vi "Blink_SDK_example.vi"() -> ()   [LabVIEW 2010]
uses:
  Blink_C_wrapper.dll
  ImageGen.dll
panel:
  out "ImgData 2":u8[](array[numeric])
  in  "Wait Timer":dbl
  out "Use External Triggers":bool
  out "BoardNum":i32
  out "ImgData":u8[](array[numeric])
  # "PCIe  LabVIEWSDK"
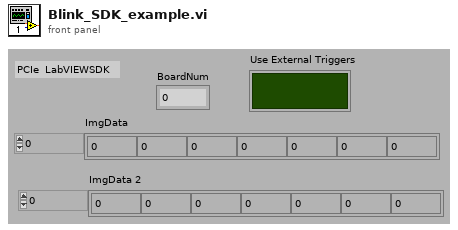
[diagram p1: front panel]
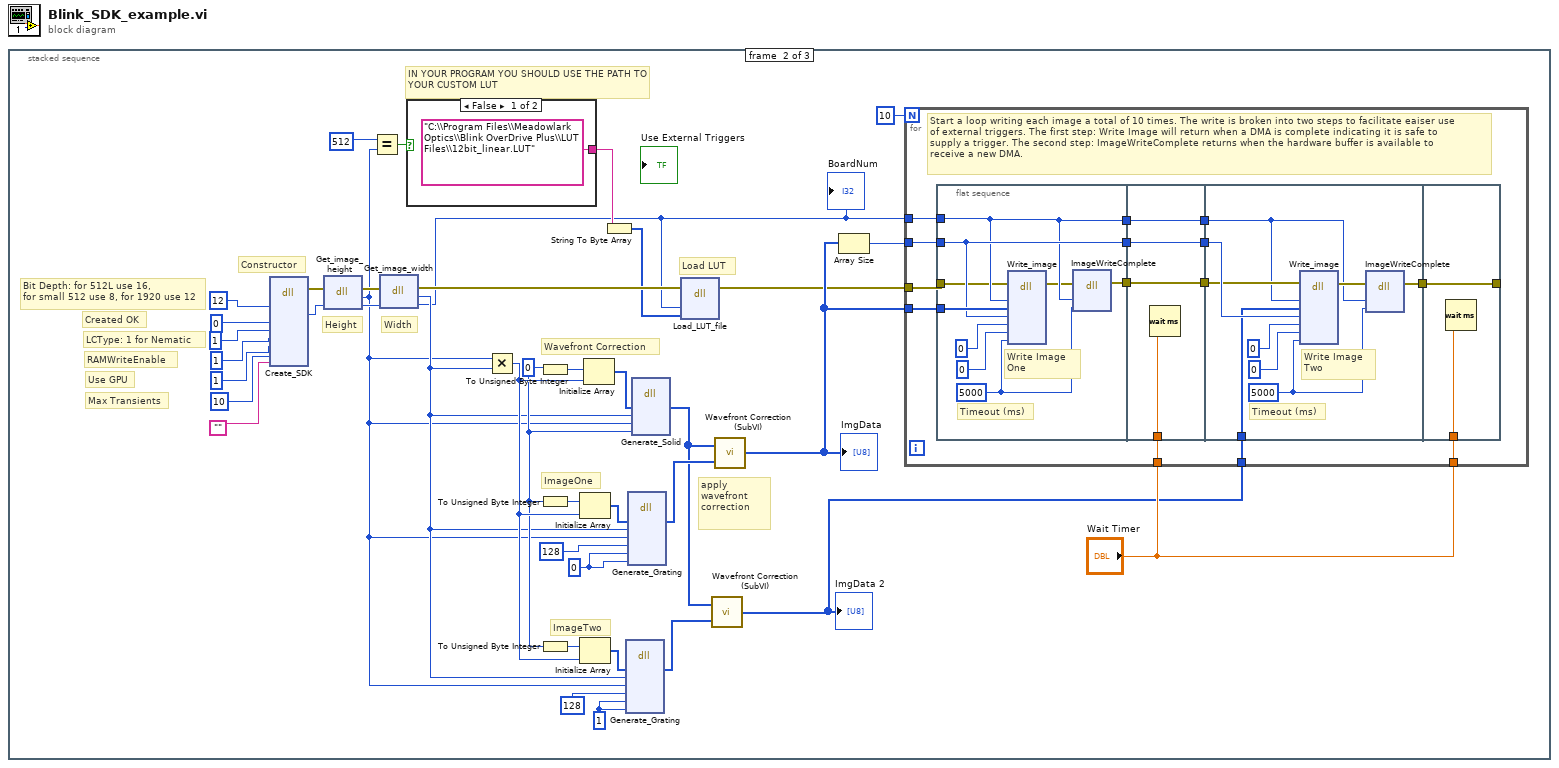
[diagram p0: block diagram]
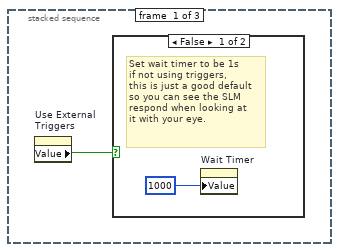
[diagram p2: hidden frame]
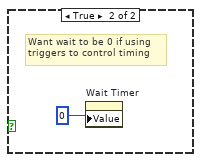
[diagram p3: hidden frame]
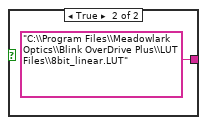
[diagram p4: hidden frame]
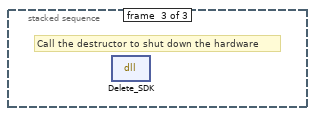
[diagram p5: hidden frame]
diagram:
  n1 = stacked-sequence {
    frame #0 {
      n2 = property on="Use External \nTriggers" class="Bool (strict)"() -> ("Value"=w1:bool)  [unwired: 2 in, 2 out]
      n3 = case shown="False" w1 {
        frame False {
          # "Set wait timer to be 1s \nif not using triggers,\nthis is just a good default \nso you can see the SLM \nrespond when looking at \nit with your eye."
          n4 = property on="Wait Timer" class="DigNum (strict)"("Value"=1000) -> ()  [unwired: 2 in, 2 out]
        }
        frame True {
          # "Want wait to be 0 if using \ntriggers to control timing"
          n5 = property on="Wait Timer" class="DigNum (strict)"("Value"=0) -> ()  [unwired: 2 in, 2 out]
        }
      }
    }
    frame #1 {
      w20 = 1
      w22 = 0
      w25 = 0
      # "IN YOUR PROGRAM YOU SHOULD USE THE PATH TO YOUR CUSTOM LUT"
      # "Load LUT"
      # "ImageTwo"
      # "ImageOne"
      # "Wavefront Correction"
      # "Width"
      # "Height"
      # "apply wavefront\ncorrection"
      # "Created OK"
      # "Max Transients"
      # "Use GPU"
      # "RAMWriteEnable"
      # "Bit Depth: for 512L use 16, \nfor small 512 use 8, for 1920 use 12"
      # "LCType: 1 for Nematic"
      # "Constructor"
      n6 = dll-call lib="C:/Program Files/Meadowlark Optics/Blink OverDrive Plus/SDK/Blink_C_wrapper.dll" fn="Create_SDK"("SLM_bit_depth"=12, "constructed_ok"=0, "is_nematic_type"=1, "RAM_write_enable"=1, "use_GPU_if_available"=1, "max_transient_frames"=10, "static_regional_lut_file"="") -> (error out=w5:errorcluster, "n_boards_found"=w4:u64)  [unwired: 12 in, 1 out]
      n7 = dll-call lib="C:/Program Files/Meadowlark Optics/Blink OverDrive Plus/SDK/Blink_C_wrapper.dll" fn="Get_image_height"(error in=w5, "Board"=w4) -> (error out=w31:errorcluster, "return type"=w9:i32, "Board"=w32:u32)  [unwired: 2 in, 1 out]
      n8 = Equal?(x=512, y=w9) -> (x = y?=w11:bool)
      n9 = dll-call lib="C:/Program Files/Meadowlark Optics/Blink OverDrive Plus/SDK/Blink_C_wrapper.dll" fn="Get_image_width"(error in=w31, "Board"=w32) -> (error out=w12:errorcluster, "return type"=w18:i32, "Board"=w6:u32)  [unwired: 2 in, 1 out]
      "BoardNum" <- w6
      n10 = case shown="False" w11 {
        tunnel: ["C:\\Program Files\\Meadowlark Optics\\Blink OverDrive Plus\\LUT Files\\12bit_linear.LUT" "C:\\Program Files\\Meadowlark Optics\\Blink OverDrive Plus\\LUT Files\\8bit_linear.LUT"] -> w8
        frame False {
        }
        frame True {
        }
      }
      n11 = Multiply(x=w9, y=w18) -> (x*y=w30:i32)
      n12 = To Unsigned Byte Integer(number=w25) -> (unsigned 8bit integer=w29:u8)
      n13 = To Unsigned Byte Integer(number=w25) -> (unsigned 8bit integer=w27:u8)
      n14 = To Unsigned Byte Integer(number=w25) -> (unsigned 8bit integer=w26:u8)
      n15 = Initialize Array(w27, w30) -> (w24:u8[])
      n16 = Initialize Array(w26, w30) -> (w21:u8[])
      n17 = Initialize Array(w29, w30) -> (w28:u8[])
      n18 = String To Byte Array(string=w8) -> (unsigned byte array=w7:u8[])
      n19 = dll-call lib="C:/Program Files/Meadowlark Optics/Blink OverDrive Plus/SDK/ImageGen.dll" fn="Generate_Grating"("Array"=w21, "Width"=w18, "Height"=w9, "Period"=128, "Increasing"=w20, "Horizontal"=w20) -> ("Array"=w15:u8[])  [unwired: 9 in, 2 out]
      n20 = dll-call lib="C:/Program Files/Meadowlark Optics/Blink OverDrive Plus/SDK/ImageGen.dll" fn="Generate_Grating"("Array"=w24, "Width"=w18, "Height"=w9, "Period"=128, "Increasing"=w22, "Horizontal"=w22) -> ("Array"=w17:u8[])  [unwired: 9 in, 2 out]
      n21 = dll-call lib="C:/Program Files/Meadowlark Optics/Blink OverDrive Plus/SDK/ImageGen.dll" fn="Generate_Solid"("Array"=w28, "Width"=w18, "Height"=w9, "PixelValue"=w25) -> ("Array"=w16:u8[])  [unwired: 7 in, 2 out]
      n22 = dll-call lib="C:/Program Files/Meadowlark Optics/Blink OverDrive Plus/SDK/Blink_C_wrapper.dll" fn="Load_LUT_file"("Board"=w6, "LUTPath"=w7) -> ()  [unwired: 6 in, 2 out]
      n23 = call "Wavefront Correction (SubVI).vi"("Source Image Array"=w15, "Wavefront Correction"=w16) -> ("Corrected Image Array"=w14:u8[])
      "ImgData 2" <- w14
      n24 = call "Wavefront Correction (SubVI).vi"("Source Image Array"=w17, "Wavefront Correction"=w16) -> ("Corrected Image Array"=w13:u8[])
      "ImgData" <- w13
      n25 = Array Size(array=w13) -> (size(s)=w34:i32)
      n26 = for {
        N: 10 -> [_]
        tunnel: w6 -> [w58]
        tunnel: w13 -> [w57]
        tunnel: w34 -> [w56]
        tunnel: w14 -> [w55]
        tunnel: "Wait Timer" -> [w50]
        tunnel: "Wait Timer" -> [w49]
        tunnel: w12 -> [w45]
        # "Start a loop writing each image a total of 10 times. The write is broken into two steps to facilitate eaiser use\nof external triggers. The first step: Write Image will return when a DMA is complete indicating it is safe to \nsupply a trigger. The second step: ImageWriteComplete returns when the hardware buffer is available to \nreceive a new DMA."
        n27 = flat-sequence {
          tunnel: w58 -> [w63]
          tunnel: w57 -> [w65]
          tunnel: w56 -> [w64]
          tunnel: [w63] -> w54
          tunnel: [w64] -> w52
          tunnel: [w60] -> w47
          tunnel: w45 -> [w59]
          tunnel: w54 -> [w71]
          tunnel: [w71] -> w53
          tunnel: w52 -> [w70]
          tunnel: [w70] -> w51
          tunnel: w50 -> [w69]
          tunnel: [w68] -> w48
          tunnel: w47 -> [w68]
          tunnel: w53 -> [w73]
          tunnel: w51 -> [w78]
          tunnel: w55 -> [w77]
          tunnel: w48 -> [w76]
          tunnel: [w74] -> w46
          tunnel: w49 -> [w82]
          tunnel: [w81] -> _
          tunnel: w46 -> [w81]
          frame #0 {
            w62 = 5000
            # "Timeout (ms)"
            # "Write Image \nOne"
            n28 = dll-call lib="C:/Program Files/Meadowlark Optics/Blink OverDrive Plus/SDK/Blink_C_wrapper.dll" fn="Write_image"(error in=w59, "board"=w63, "Image"=w65, "ImageSize"=w64, "WaitForTrigger"=0, "ExternalPulse"=0, "timeout"=w62) -> (error out=w61:errorcluster)  [unwired: 9 in, 1 out]
            n29 = dll-call lib="C:/Program Files/Meadowlark Optics/Blink OverDrive Plus/SDK/Blink_C_wrapper.dll" fn="ImageWriteComplete"(error in=w61, "board"=w63, "timeout"=w62) -> (error out=w60:errorcluster)  [unwired: 5 in, 1 out]
          }
          frame #1 {
            n30 = Wait (ms)(milliseconds to wait=w69) -> ()  [unwired: 1 out]
          }
          frame #2 {
            w72 = 5000
            # "Timeout (ms)"
            # "Write Image \nTwo"
            n31 = dll-call lib="C:/Program Files/Meadowlark Optics/Blink OverDrive Plus/SDK/Blink_C_wrapper.dll" fn="Write_image"(error in=w76, "board"=w73, "Image"=w77, "ImageSize"=w78, "WaitForTrigger"=0, "ExternalPulse"=0, "timeout"=w72) -> (error out=w75:errorcluster)  [unwired: 9 in, 1 out]
            n32 = dll-call lib="C:/Program Files/Meadowlark Optics/Blink OverDrive Plus/SDK/Blink_C_wrapper.dll" fn="ImageWriteComplete"(error in=w75, "board"=w73, "timeout"=w72) -> (error out=w74:errorcluster)  [unwired: 5 in, 1 out]
          }
          frame #3 {
            n33 = Wait (ms)(milliseconds to wait=w82) -> ()  [unwired: 1 out]
          }
        }
      }
    }
    frame #2 {
      # "Call the destructor to shut down the hardware"
      n34 = dll-call lib="C:/Program Files/Meadowlark Optics/Blink OverDrive Plus/SDK/Blink_C_wrapper.dll" fn="Delete_SDK"() -> ()  [unwired: 4 in, 2 out]
    }
  }
